vi "Analog_Input_8Channels_W16I5.vi"(1 "IO":T1={"AI 0"="Mod3/AI0", "AI 1"="Mod3/AI0", "AI 2"="Mod3/AI0", "AI 3"="Mod3/AI0", "AI 4"="Mod3/AI0", "AI 5"="Mod3/AI0", "AI 6"="Mod3/AI0", "AI 7"="Mod3/AI0"}) -> (0 "Values":fxp<+/-,16,5>[](array[numeric]))   [LabVIEW 2015, in "FPGA Wizard Templates.lvlib"]
uses:
  FPGA Wizard Templates.lvlib
  <vilib>/rvi/eio/common/nirviEmuTemplateMethod_errors.vi
  <vilib>/eio/EIONode/EIONode.xnode
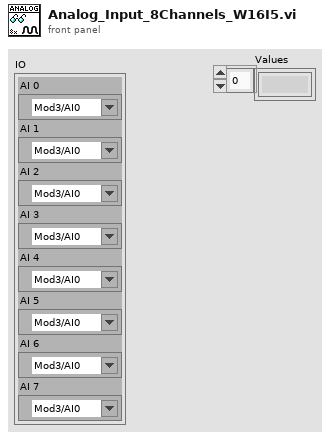
[diagram p1: front panel]
types:
  T1 = cluster{"AI 0":refnum<k21>, "AI 1":refnum<k21>, "AI 2":refnum<k21>, "AI 3":refnum<k21>, "AI 4":refnum<k21>, "AI 5":refnum<k21>, "AI 6":refnum<k21>, "AI 7":refnum<k21>}
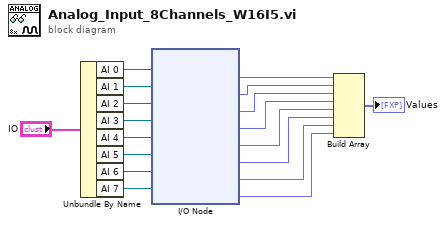
[diagram p0: block diagram]
diagram:
  n1 = Unbundle By Name("IO") -> ("AI 0"=w17:refnum<k21>, "AI 1"=w16:refnum<k21>, "AI 2"=w15:refnum<k21>, "AI 3"=w14:refnum<k21>, "AI 4"=w13:refnum<k21>, "AI 5"=w12:refnum<k21>, "AI 6"=w11:refnum<k21>, "AI 7"=w10:refnum<k21>)
  n2 = xnode "I/O Node"("FPGA I/O In"=w17, "FPGA I/O In"=w16, "FPGA I/O In"=w15, "FPGA I/O In"=w14, "FPGA I/O In"=w13, "FPGA I/O In"=w12, "FPGA I/O In"=w11, "FPGA I/O In"=w10) -> ("I/O Item"=w9:fxp<+/-,16,5>, "I/O Item"=w8:fxp<+/-,16,5>, "I/O Item"=w7:fxp<+/-,16,5>, "I/O Item"=w6:fxp<+/-,16,5>, "I/O Item"=w5:fxp<+/-,16,5>, "I/O Item"=w4:fxp<+/-,16,5>, "I/O Item"=w3:fxp<+/-,16,5>, "I/O Item"=w2:fxp<+/-,16,5>)  [unwired: 8 out]
  n3 = Build Array(w9, w8, w7, w6, w5, w4, w3, w2) -> (→"Values":fxp<+/-,16,5>[])
